vi "Timestamp to Text.vi"(7 "Local Time Offset format":bool, 8 "error in (no error)":errorcluster, 11 "Time Stamp":timestamp) -> (0 "error out":errorcluster, 3 "Timestamp (RFC3339)":string)   [LabVIEW 2019, in "JDP Timestamp.lvlib"]
doc: "Convert Timestamp to Text coresponding to RFC3339 standard format.\n\nExample:\n2020-06-25T08:50:15.123Z\n\nIf \"Local Time Offset format\" is true, then this example would format as:\n2020-06-25T09:50:15.123+01:00\n\nRFC3339--> https://tools.ietf.org/html/rfc3339"
uses:
  JDP Timestamp.lvlib
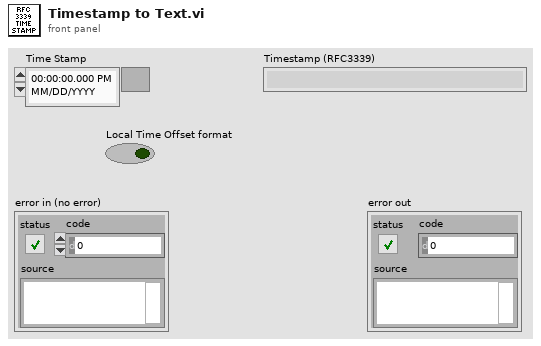
[diagram p1: front panel]
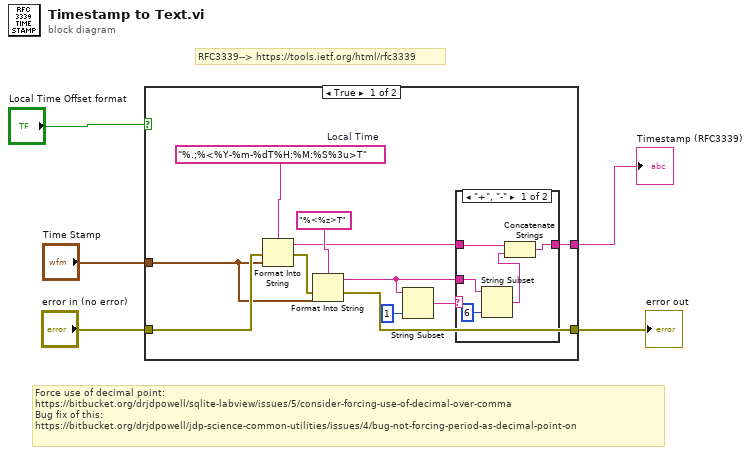
[diagram p0: block diagram]
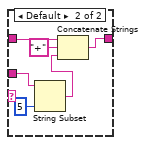
[diagram p2: hidden frame]
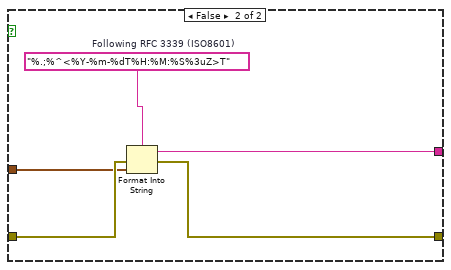
[diagram p3: hidden frame]
diagram:
  # "RFC3339--> https://tools.ietf.org/html/rfc3339"
  # "Force use of decimal point:\nhttps://bitbucket.org/drjdpowell/sqlite-labview/issues/5/consider-forcing-use-of-decimal-over-comma\nBug fix of this: \nhttps://bitbucket.org/drjdpowell/jdp-science-common-utilities/issues/4/bug-not-forcing-period-as-decimal-point-on"
  n1 = case shown="True" "Local Time Offset format" {
    tunnel: [w12 w32] -> w5
    tunnel: "error in (no error)" -> [w16 w31]
    tunnel: [w6 w30] -> w3
    tunnel: "Time Stamp" -> [w14 w29]
    frame True {
      w15 = "%.;%<%Y-%m-%dT%H:%M:%S%3u>T"  # Local Time
      n2 = Format Into String(format string=w15, error in=w16, w14) -> (resulting string=w8:string, error out=w13:errorcluster)  [unwired: 1 in]
      n3 = Format Into String(format string="%<%z>T", error in=w13, w14) -> (resulting string=w7:string, error out=w12:errorcluster)  [unwired: 1 in]
      n4 = String Subset(string=w7, length (rest)=1 ("length (rest)")) -> (substring=w9:string)  [unwired: 1 in]
      n5 = case shown="\"+\", \"-\"" w9 {
        tunnel: w8 -> [w21 w27]
        tunnel: w7 -> [w18 w24]
        tunnel: [w20 w26] -> w6
        frame "+", "-" {
          n6 = String Subset(string=w18, length (rest)=6 ("length (rest)")) -> (substring=w17:string)  [unwired: 1 in]
          n7 = Concatenate Strings(w21, w17) -> (w20:string)
        }
        frame Default {
          n8 = String Subset(string=w24, length (rest)=5 ("length (rest)")) -> (substring=w23:string)  [unwired: 1 in]
          n9 = Concatenate Strings(w27, "+" ("string"), w23) -> (w26:string)
        }
      }
    }
    frame False {
      w28 = "%.;%^<%Y-%m-%dT%H:%M:%S%3uZ>T"  # Following RFC 3339 (ISO8601)
      n10 = Format Into String(format string=w28, error in=w31, w29) -> (resulting string=w30:string, error out=w32:errorcluster)  [unwired: 1 in]
    }
  }
  "error out" <- w5
  "Timestamp (RFC3339)" <- w3
